vi "Unsubscribe from Context.vi"(8 "error in (no error)":errorcluster, 9 "Context":T1, 10 "Subscriber Enq":refnum<class "Message Enqueuer.lvclass">, 11 "Publisher Actor in":refnum<class "Publisher Actor.lvclass">) -> (0 "error out":errorcluster, 3 "Publisher Actor out":refnum<class "Publisher Actor.lvclass">)   [LabVIEW 2021, in "Publisher Actor.lvclass"]
uses:
  Publisher Actor.lvclass
  Context.ctl
  <vilib>/ActorFramework/Message Enqueuer/Message Enqueuer.lvclass
  Publisher Actor.lvclass/Publisher Actor.ctl
  24312427-c68e-485d-b05f-91bbb587ca92.vi
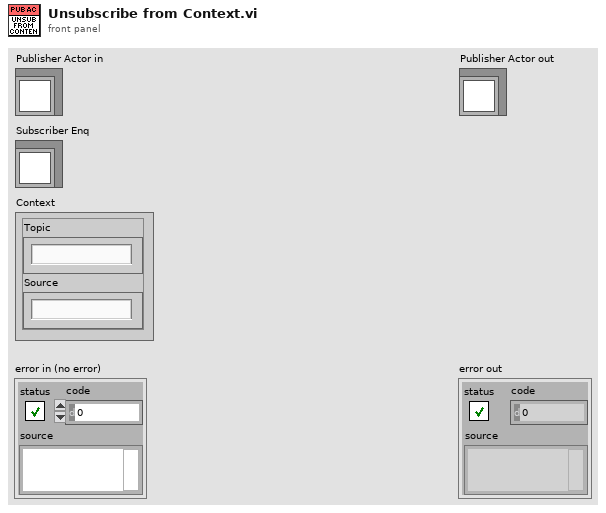
[diagram p1: front panel]
types:
  T1 = typedef "Context.ctl" = cluster{"Topic":string, "Source":string}
  T2 = map{T1, set{refnum<class "Message Enqueuer.lvclass">}}
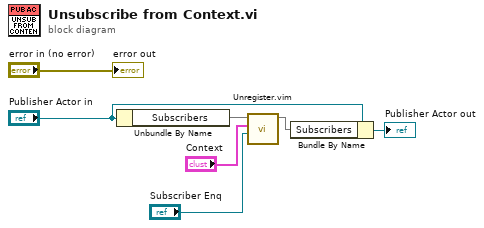
[diagram p0: block diagram]
diagram:
  n1 = Unbundle By Name("Publisher Actor in") -> ("Subscribers"=w6:T2)
  n2 = call "Unregister.vim"("set element"="Subscriber Enq", "key"="Context", "map in"=w6) -> ("map out"=w7:T2)  [unwired: 6 in, 2 out]
  n3 = Bundle By Name(cluster="Publisher Actor in", "Subscribers"=w7) -> (→"Publisher Actor out":refnum<class "Publisher Actor.lvclass">)
  "error out" <- "error in (no error)"
